vi "VLC - Play Stream&Snapshot&speed.vi"(5 "Media Source":string="rtsp://admin:admin@192.168.1.108/cam/realmonitor?channel=1&subtype=1", 7 "Script":string, 11 "error in (no error)":errorcluster) -> (15 "error out":errorcluster)   [LabVIEW 2016]
uses:
  System.Windows.Forms
  <vilib>/Utility/sysdir.llb/System Directory Type.ctl
  <vilib>/picture/picture.llb/imagedata.ctl
  USER32.DLL
panel:
  out "VLC Istance pointer":i32
  in  "PictureBox 2":refnum<k24>(container)
  out "hWnd 3":u32
  out "error out 2":errorcluster
  out "hWnd 2":u32
  out "hWnd":u32
  in  "Image 2":T1(plugin-control)
  in  "2D Picture":picture
  out "Image":T1(plugin-control)
  out "return type":i32
  out "speed":dbl
  in  "Snap":bool
  # "rtsp://admin:admin@192.168.1.108/cam/realmonitor?channel=1&subtype=1"
  # "rtsp://admin:gamma2018@84.253.163.35:554/cam/realmonitor?channel=1&subtype=1"
  # "the target computer for the application must have the .NET Framework 4.0 installed."
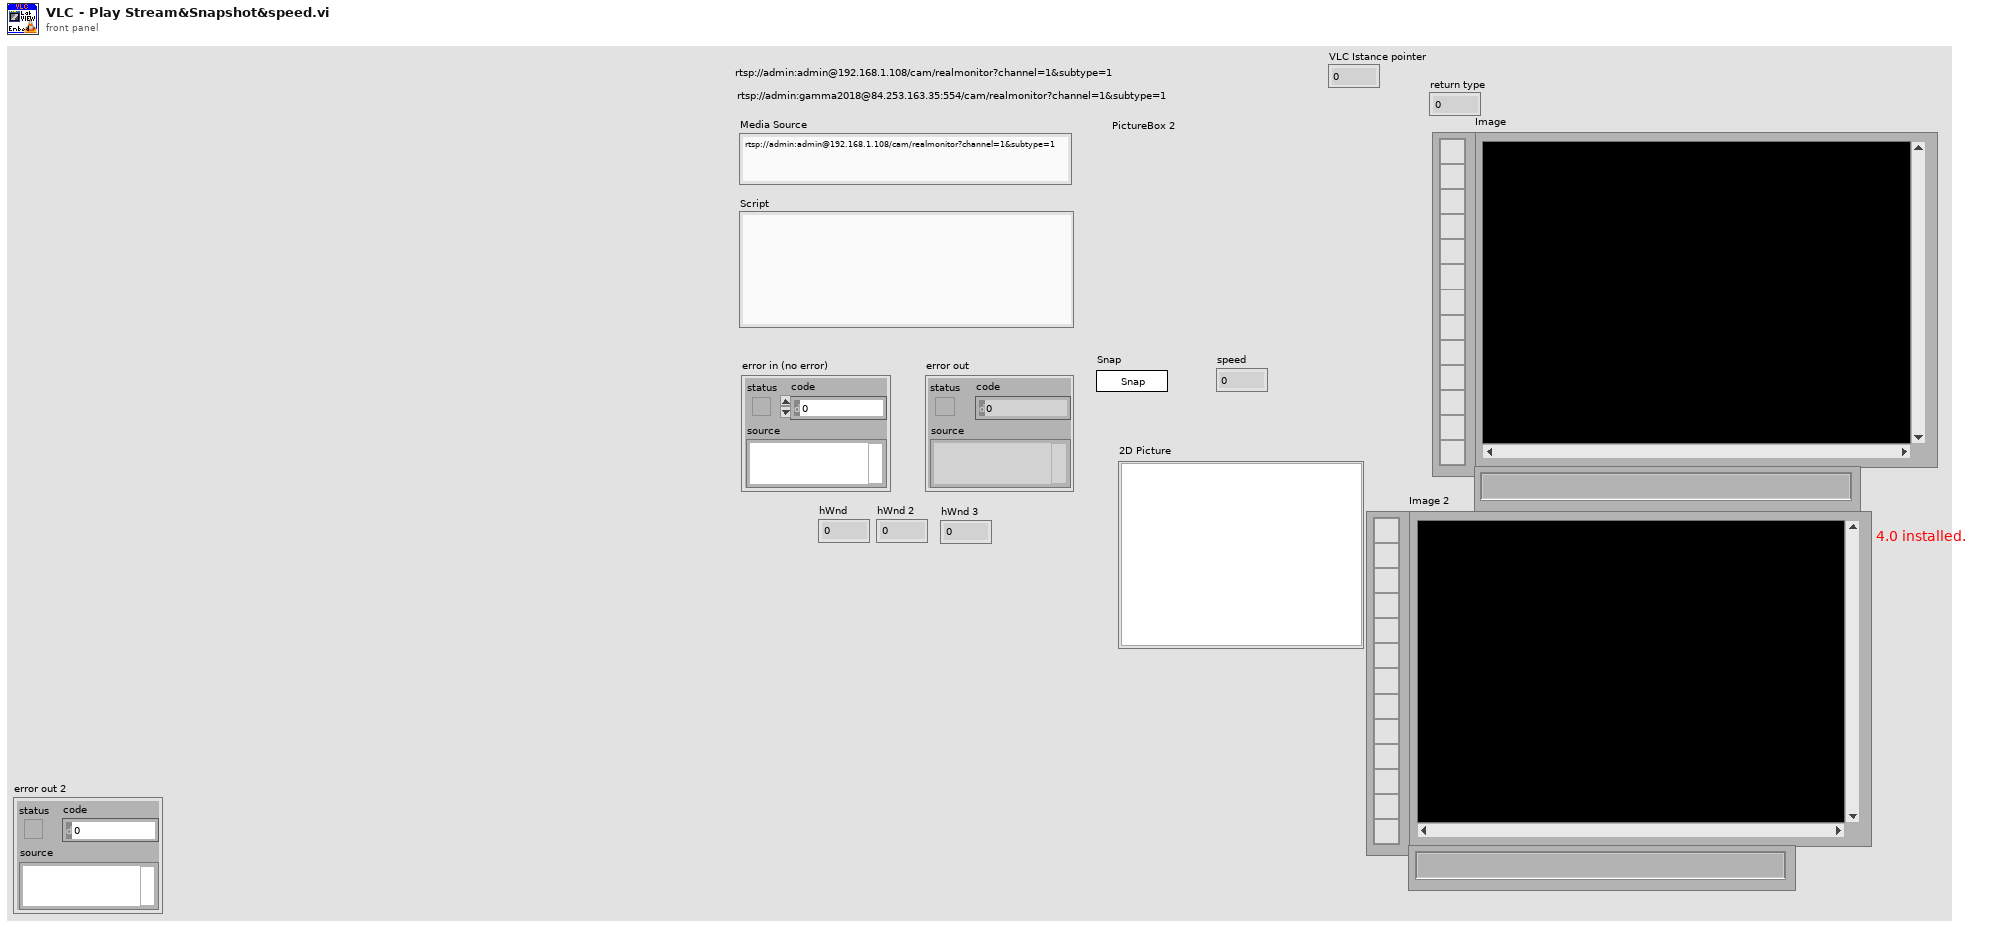
[diagram p1: front panel]
types:
  T1 = typedef "IMAQ Image.ctl" = refnum<image>
  T2 = typedef "System Directory Type.ctl" = i32
  T3 = typedef "imagedata.ctl" = cluster{"image type":i32, "image depth":i32, "image":u8[], "mask":u8[], "colors":u32[], "Rectangle":cluster{"left":i16, "top":i16, "right":i16, "bottom":i16}}
  T4 = typedef "Image Type" = u32
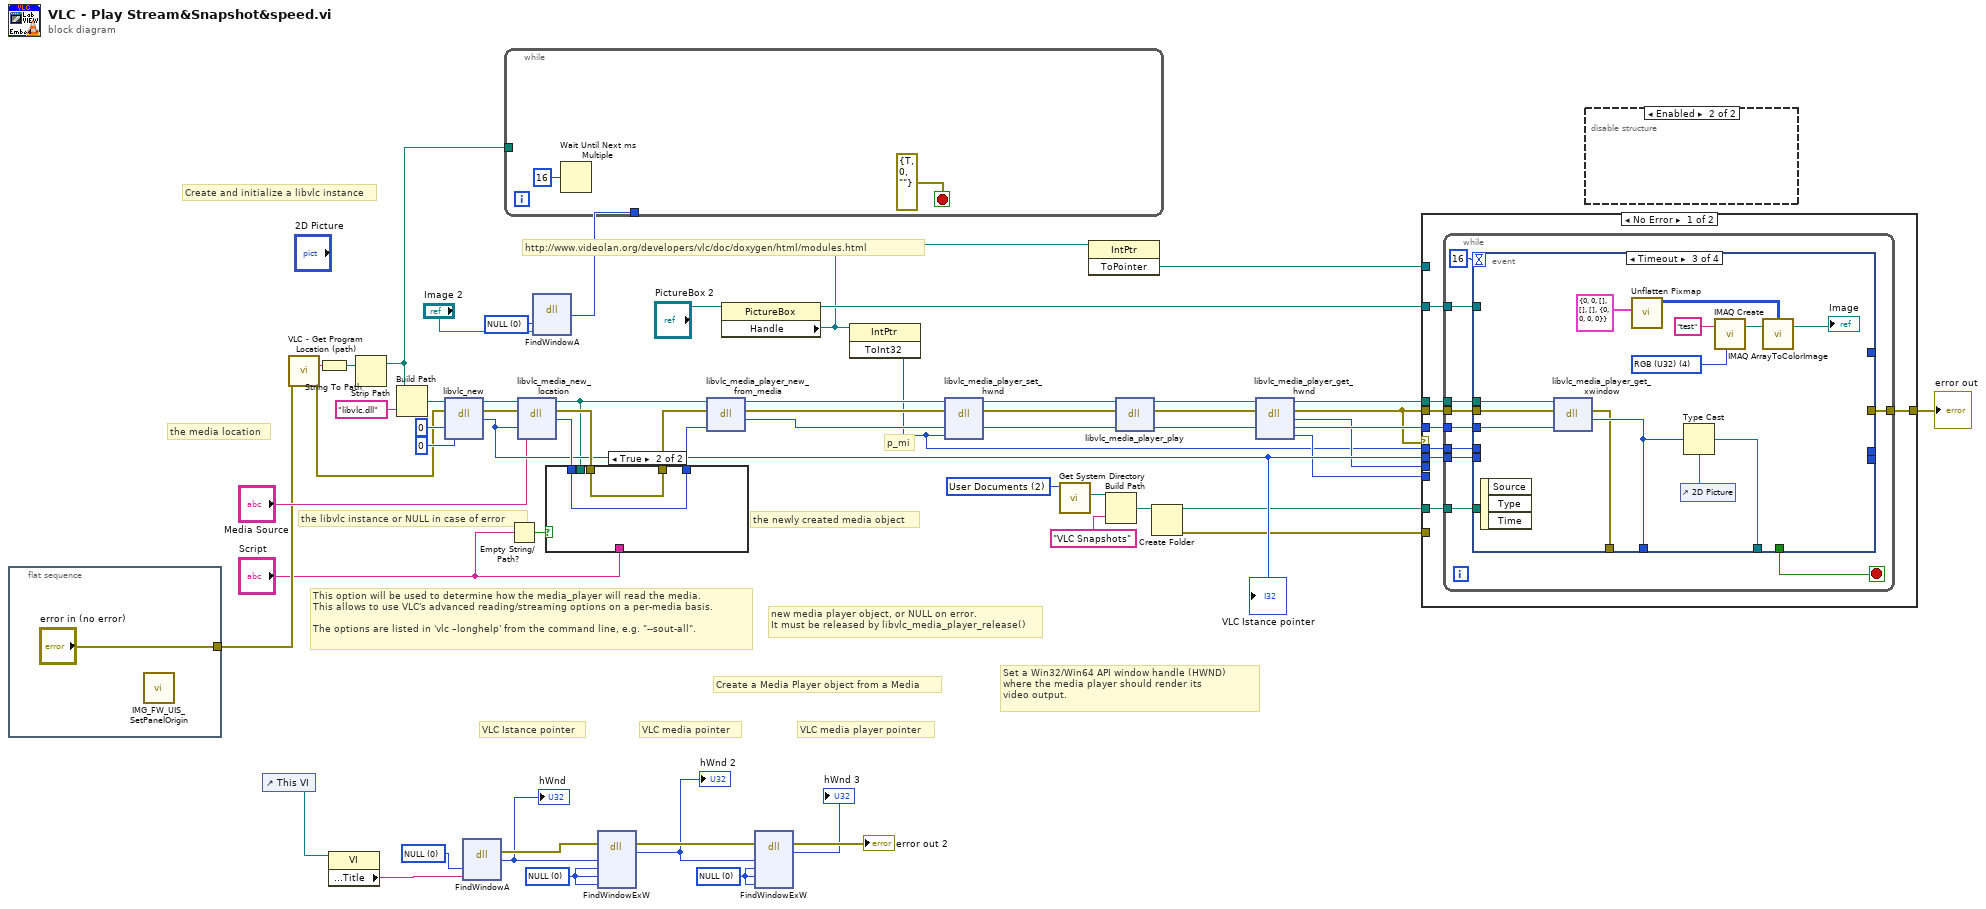
[diagram p0: block diagram]
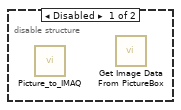
[diagram p2: hidden frame]
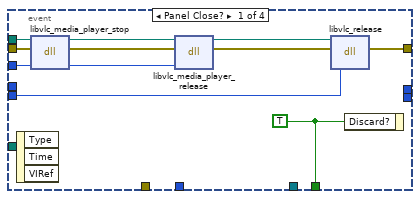
[diagram p3: hidden frame]
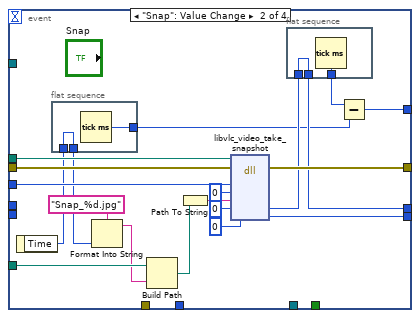
[diagram p4: hidden frame]
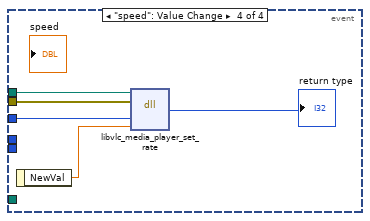
[diagram p5: hidden frame]
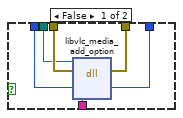
[diagram p7: hidden frame]
diagram:
  w10 = 0 items=["NULL"]
  w14 = 0 items=["NULL"]
  w16 = 0 items=["NULL"]
  w26 = 0 items=["NULL"]
  w36 = T2 2 items=["User Home"=0, "User Desktop"=1, "User Documents"=2, "User Application Data"=3, "User Preferences"=4, "User Temporary"=5, "Public Documents"=6, "Public Application Data"=7, "Public Preferences"=8, "Public Cache"=13, "System Core Libraries"=9, "System Installed Libraries"=10, "Application Files"=11, "Boot Volume Root"=12] ("system directory type")
  # "VLC media player pointer"
  # "VLC media pointer"
  # "VLC Istance pointer"
  # "p_mi"
  # "Set a Win32/Win64 API window handle (HWND) \nwhere the media player should render its \nvideo output."
  # "new media player object, or NULL on error. \nIt must be released by libvlc_media_player_release()"
  # "Create a Media Player object from a Media"
  # "This option will be used to determine how the media_player will read the media. \nThis allows to use VLC's advanced reading/streaming options on a per-media basis.\n\nThe options are listed in 'vlc –longhelp' from the command line, e.g. \"--sout-all\"."
  # "the newly created media object"
  # "the media location"
  # "Create and initialize a libvlc instance"
  # "the libvlc instance or NULL in case of error"
  # "http://www.videolan.org/developers/vlc/doc/doxygen/html/modules.html"
  n1 = flat-sequence {
    tunnel: ["error in (no error)"] -> w42
    frame #0 {
      n2 = call "IMG_FW_UIS_SetPanelOrigin.vi"() -> ()  [unwired: 11 in, 1 out]
    }
  }
  n3 = control-ref of="This VI"() -> (w6:refnum<vi>)
  n4 = call "VLC - Get Program Location (path).vi"("error in (no error)"=w42) -> ("VLC path"=w47:string, "error out"=w41:errorcluster)  [unwired: 13 in]
  n5 = String To Path(string=w47) -> (path=w46:path)
  n6 = property class="VI"(reference=w6) -> ("Front Panel Window:Title"=w15:string)  [unwired: 1 in, 2 out]
  n7 = Strip Path(path=w46) -> (stripped path=w27:path)  [unwired: 1 out]
  n8 = Build Path(base path=w27, name or relative path="libvlc.dll") -> (appended path=w44:path)
  n9 = dll-call lib="C:/Program Files (x86)/VideoLAN/VLC/libvlc.dll" fn="libvlc_new"(path in=w44, error in=w41, "argc"=i16 0, "argv"=u8 0) -> (path out=w50:path, error out=w53:errorcluster, "return type"=w56:i32)  [unwired: 3 in]
  "VLC Istance pointer" <- w56
  n10 = dll-call lib="USER32.DLL" fn="FindWindowA" label="FindWindow"("lpszClassName"=w16, "lpszWindowName"=w15) -> (error out=w13:errorcluster, "hWnd"=w7:u32)  [unwired: 5 in, 1 out]
  "hWnd" <- w7
  n11 = Empty String/Path?(string/path="Script") -> (empty?=w39:bool)
  n12 = dll-call lib="C:/Program Files (x86)/VideoLAN/VLC/libvlc.dll" fn="libvlc_media_new_location"(path in=w50, error in=w53, "p_instance"=w56, "path"="Media Source") -> (path out=w37:path, error out=w57:errorcluster, "return type"=w58:i32)  [unwired: 3 in]
  n13 = dll-call lib="USER32.DLL" fn="FindWindowA" label="FindWindow"("lpszClassName"=w26, "lpszWindowName"="Image 2") -> ("hWnd"=w24:u32)  [unwired: 5 in, 2 out]
  n14 = while {
    tunnel: w27 -> [_]
    tunnel: w24 -> [_]
    stop <- errorcluster {"status"=TRUE, "code"=0, "source"=""} ("error IO") stop-if-true
    n15 = Wait Until Next ms Multiple(millisecond multiple=u32 16) -> ()  [unwired: 1 out]
  }
  n16 = case shown="True" w39 {
    tunnel: w57 -> [w69 w71]
    tunnel: w58 -> [w68 w70]
    tunnel: [w67 w70] -> w59
    tunnel: [w66 w71] -> w60
    tunnel: "Script" -> [w65 _]
    tunnel: w37 -> [w64 _]
    frame False {
      n17 = dll-call lib="C:/Program Files (x86)/VideoLAN/VLC/libvlc.dll" fn="libvlc_media_add_option"(path in=w64, error in=w69, "p_md"=w68, "ppsz_options"=w65) -> (error out=w66:errorcluster, "p_md"=w67:i32)  [unwired: 3 in, 1 out]
    }
    frame True {
    }
  }
  n18 = dll-call lib="user32.dll" fn="FindWindowExW" label="FindWindowEx"(error in=w13, "hwndParent"=w7, "hwndChildAfter"=w14, "lpszClassName"=w14, "lpszWindowName"=w14) -> (error out=w12:errorcluster, "hWnd"=w11:u32)  [unwired: 6 in, 1 out]
  "hWnd 2" <- w11
  n19 = dll-call lib="C:/Program Files (x86)/VideoLAN/VLC/libvlc.dll" fn="libvlc_media_player_new_from_media"(path in=w37, error in=w60, "p_md"=w59) -> (path out=w49:path, error out=w55:errorcluster, "return type"=w54:i32)  [unwired: 2 in]
  n20 = property class="PictureBox"(reference="PictureBox 2") -> (reference out=w29:refnum<k24>, "Handle"=w4:refnum<k24>)  [unwired: 1 in, 1 out]
  n21 = dll-call lib="user32.dll" fn="FindWindowExW" label="FindWindowEx"(error in=w12, "hwndParent"=w11, "hwndChildAfter"=w10, "lpszClassName"=w10, "lpszWindowName"=w10) -> (error out=→"error out 2":errorcluster, "hWnd"=→"hWnd 3":u32)  [unwired: 6 in, 1 out]
  n22 = invoke class="IntPtr" method="ToInt32"(reference=w4) -> ("ToInt32"=w1:i32)  [unwired: 2 in, 2 out]
  n23 = dll-call lib="C:/Program Files (x86)/VideoLAN/VLC/libvlc.dll" fn="libvlc_media_player_set_hwnd"(path in=w49, error in=w55, "p_mi"=w54, "drawable"=w1) -> (path out=w48:path, error out=w28:errorcluster, "p_mi"=w30:i32)  [unwired: 3 in]
  n24 = call <vilib>:"Get System Directory.vi"("system directory type"=w36) -> ("system directory"=w35:path)  [unwired: 10 in]
  n25 = invoke class="IntPtr" method="ToPointer"(reference=w4) -> ("ToPointer"=w3:refnum<k24>)  [unwired: 2 in, 2 out]
  n26 = Build Path(base path=w35, name or relative path="VLC Snapshots") -> (appended path=w33:path)
  n27 = dll-call lib="C:/Program Files (x86)/VideoLAN/VLC/libvlc.dll" fn="libvlc_media_player_play"(path in=w48, error in=w28, "p_mi"=w30) -> (path out=w23:path, error out=w18:errorcluster, "p_mi"=w21:i32)  [unwired: 2 in]
  n28 = Create Folder(path (use dialog)=w33) -> (created path=w32:path, error out=w31:errorcluster)  [unwired: 2 in, 1 out]
  n29 = dll-call lib="C:/Program Files (x86)/VideoLAN/VLC/libvlc.dll" fn="libvlc_media_player_get_hwnd"(path in=w23, error in=w18, "p_mi"=w21) -> (path out=w22:path, error out=w17:errorcluster, "return type"=w2:i32, "p_mi"=w20:i32, "drawable"=w19:i32)  [unwired: 2 in]
  n30 = case shown="No Error" w17 {
    tunnel: w56 -> [w79 _]
    tunnel: w20 -> [w78 _]
    tunnel: w17 -> [w77 w143]
    tunnel: w22 -> [w76 _]
    tunnel: [w75 w143] -> w38
    tunnel: w32 -> [w74 _]
    tunnel: w31 -> [_ _]
    tunnel: w29 -> [w73 _]
    tunnel: w19 -> [_ _]
    tunnel: w3 -> [_ _]
    tunnel: w2 -> [_ _]
    tunnel: w1 -> [w72 _]
    frame No Error {
      n31 = while {
        tunnel: w79 -> [w89]
        tunnel: w78 -> [w88]
        tunnel: w77 -> [w87]
        tunnel: w76 -> [w86]
        tunnel: [w85] -> w75
        tunnel: w74 -> [w83]
        tunnel: w73 -> [w81]
        tunnel: w72 -> [w80]
        stop <- w84 stop-if-true
        n32 = event shown="[2] Timeout" {
          selector: _ -> [_ _ _ _]
          dyn-events: _ -> [_ _ _ _]
          timeout: 16 -> [_ _ _ _]
          tunnel: w87 -> [w100 w115 w129 w141]
          tunnel: w88 -> [w99 w113 w125 w140]
          tunnel: w89 -> [w95 _ _ _]
          tunnel: w86 -> [w94 w116 w126 w142]
          tunnel: [w91 w114 _ _] -> w85
          tunnel: [w90 _ _ _] -> w84
          tunnel: w83 -> [_ w111 _ _]
          tunnel: w81 -> [_ _ _ _]
          tunnel: [_ _ w131 _] -> _
          tunnel: [_ _ w130 _] -> _
          tunnel: [_ w104 _ _] -> _
          tunnel: [_ w106 _ _] -> _
          tunnel: [_ w101 _ _] -> _
          tunnel: w80 -> [_ _ _ _]
          tunnel: [_ _ w128 _] -> _
          event Panel Close? {
            w90 = TRUE ("Discard?")
            n33 = event-data() -> ()  [unwired: 1 in, 3 out]
            n34 = dll-call lib="C:/Program Files (x86)/VideoLAN/VLC/libvlc.dll" fn="libvlc_media_player_stop"(path in=w94, error in=w100, "p_mi"=w99) -> (path out=w93:path, error out=w98:errorcluster, "p_mi"=w97:i32)  [unwired: 2 in]
            n35 = dll-call lib="C:/Program Files (x86)/VideoLAN/VLC/libvlc.dll" fn="libvlc_media_player_release"(path in=w93, error in=w98, "p_mi"=w97) -> (path out=w92:path, error out=w96:errorcluster)  [unwired: 3 in]
            n36 = dll-call lib="C:/Program Files (x86)/VideoLAN/VLC/libvlc.dll" fn="libvlc_release"(path in=w92, error in=w96, "p_instnace"=w95) -> (error out=w91:errorcluster)  [unwired: 3 in, 1 out]
            n37 = event-data("Discard?"=w90) -> ()  [unwired: 1 in, 1 out]
          }
          event "Snap": Value Change {
            n38 = event-data() -> ("Time"=w108:u32)  [unwired: 1 in]
            n39 = flat-sequence {
              tunnel: [w124] -> w107
              tunnel: w108 -> [w124]
              tunnel: [w123] -> w102
              frame #0 {
                n40 = Tick Count (ms)() -> (millisecond timer value=w123:u32)
              }
            }
            n41 = Format Into String(format string="Snap_%d.jpg", w107) -> (resulting string=w110:string)  [unwired: 2 in, 1 out]
            n42 = Build Path(base path=w111, name or relative path=w110) -> (appended path=w109:path)
            n43 = Path To String(path=w109) -> (string=w118:string)
            n44 = dll-call lib="C:/Program Files (x86)/VideoLAN/VLC/libvlc.dll" fn="libvlc_video_take_snapshot"(path in=w116, error in=w115, "p_mi"=w113, "num"=u32 0, "psz_filepath"=w118, "i_width"=u32 0, "i_height"=u32 0) -> (error out=w114:errorcluster, "i_width"=w105:u32, "i_height"=w106:u32)  [unwired: 5 in, 1 out]
            n45 = flat-sequence {
              tunnel: [w122] -> w104
              tunnel: w105 -> [w122]
              tunnel: [w121] -> w103
              frame #0 {
                n46 = Tick Count (ms)() -> (millisecond timer value=w121:u32)
              }
            }
            n47 = Subtract(x=w103, y=w102) -> (x-y=w101:u32)
          }
          event Timeout {
            w134 = T4 4 items=["Grayscale (U8)", "Grayscale (I16)", "Grayscale (SGL)", "Complex (CSG)", "RGB (U32)", "HSL (U32)", "RGB (U64)", "Grayscale (U16)"] ("Image Type")
            n48 = event-data() -> ()  [unwired: 1 in, 3 out]
            n49 = dll-call lib="C:/Program Files (x86)/VideoLAN/VLC/libvlc.dll" fn="libvlc_media_player_get_xwindow"(path in=w126, error in=w129, "p_mi"=w125) -> (error out=w128:errorcluster, "return type"=w131:i32)  [unwired: 2 in, 1 out]
            n50 = call <vilib>:"Unflatten Pixmap.vi"("image data"=T3 {"image type"=0, "image depth"=0, "image"=[], "mask"=[], "colors"=[], "Rectangle"={"left"=0, "top"=0, "right"=0, "bottom"=0}}) -> ("24-bit pixmap"=w133:u32[][])  [unwired: 4 in, 6 out]
            n51 = control-ref of="2D Picture"() -> (w127:refnum<vi>)
            n52 = Type Cast(type=w127, x=w131) -> (*(type *) &x=w130:refnum<vi>)
            n53 = call "IMAQ Create"("Image Name"="test", "Image Type"=w134) -> ("New Image"=w136:T1)  [unwired: 3 in, 1 out]
            n54 = call "IMAQ ArrayToColorImage"("Image Pixels (U32)"=w133, "Image"=w136) -> ("Image Out"=→"Image":T1)  [unwired: 3 in, 1 out]
          }
          event "speed": Value Change {
            n55 = event-data() -> ("NewVal"=w139:dbl)  [unwired: 1 in]
            n56 = dll-call lib="C:/Program Files (x86)/VideoLAN/VLC/libvlc.dll" fn="libvlc_media_player_set_rate"(path in=w142, error in=w141, "p_mi"=w140, "rate"=w139) -> ("return type"=→"return type":i32)  [unwired: 3 in, 2 out]
          }
        }
      }
    }
    frame Error {
    }
  }
  "error out" <- w38
  n57 = disable-structure shown="Enabled" {
    frame Disabled {
      n58 = call "Picture_to_IMAQ.vi"() -> ()  [unwired: 11 in, 1 out]
      n59 = call "Get Image Data From PictureBox.vi"() -> ()  [unwired: 9 in, 3 out]
    }
    frame Enabled {
    }
  }
